vi "GET_ActiveData.vi"(8 "error in (no error)":errorcluster, 11 "FakedArray in":refnum<class "FakedArray.lvclass">) -> (0 "error out":errorcluster, 1 "Active Data []":i32[](array[numeric]), 2 "Path & Icon":T1, 3 "FakedArray out":refnum<class "FakedArray.lvclass">, 4 "Locked Layer":i32, 6 "Layer Locked?":bool)   [LabVIEW 2021, in "FakedArray.lvclass"]
uses:
  <resource>/plugins/NIIconEditor/Class/FakedArray/FakedArray.lvclass
  <vilib>/LabVIEW Icon API/lv_icon/Controls/Graphic.ctl
  <resource>/plugins/NIIconEditor/Class/FakedArray/FakedArray.lvclass/FakedArray.ctl
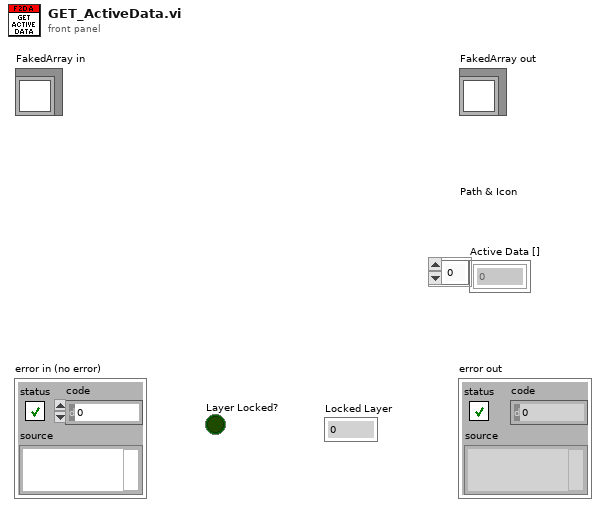
[diagram p1: front panel]
types:
  T1 = typedef "Graphic.ctl" = cluster{"Rectangle":cluster{"left":i16, "top":i16, "right":i16, "bottom":i16}, "Path":path, "Image":picture, "Filter":string, "FileName":string}
  T2 = typedef "ToMoreSpecific_Faked2DArray.ctl" = enum16{"Framework Templates", "Layer List"}
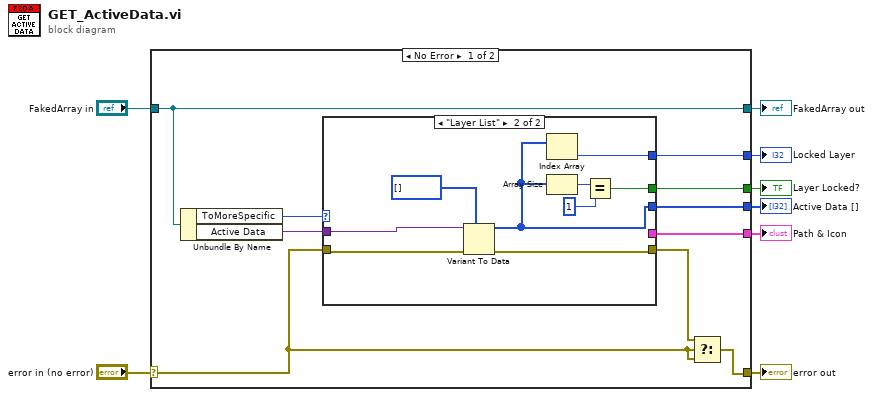
[diagram p0: block diagram]
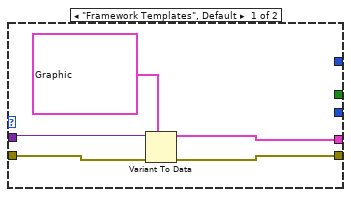
[diagram p2: hidden frame]
diagram:
  n1 = case shown="No Error" "error in (no error)" {
    selector: "error in (no error)" -> [w14 w34]
    tunnel: [w12 w34] -> w7
    tunnel: [w18 w33] -> w5
    tunnel: "FakedArray in" -> [w18 w33]
    tunnel: [w15 _] -> w4
    tunnel: [w11 _] -> w3
    tunnel: [w10 _] -> w2
    tunnel: [w9 _] -> w1
    frame No Error {
      n2 = Unbundle By Name(w18) -> ("ToMoreSpecific"=w17:T2, "Active Data"=w16:variant)
      n3 = case shown="\"Layer List\"" w17 {
        tunnel: w16 -> [w23 w32]
        tunnel: w14 -> [w22 w31]
        tunnel: [w21 w30] -> w13
        tunnel: [w19 _] -> w15
        tunnel: [_ w25] -> w11
        tunnel: [_ w26] -> w10
        tunnel: [_ w24] -> w9
        frame "Framework Templates", Default {
          n4 = Variant To Data(error in=w22, type=T1 {"Rectangle"={"left"=0, "top"=0, "right"=0, "bottom"=0}, "Path"=path "", "Image"=bytes[0], "Filter"="", "FileName"=""} ("Path & Icon"), Variant=w23) -> (data=w19:T1, error out=w21:errorcluster)
        }
        frame "Layer List" {
          n5 = Variant To Data(error in=w31, type=i32[] [], Variant=w32) -> (data=w25:i32[], error out=w30:errorcluster)
          n6 = Index Array(array=w25) -> (element=w24:i32)  [unwired: 1 in]
          n7 = Array Size(array=w25) -> (size(s)=w28:i32)
          n8 = Equal?(x=w28, y=1) -> (x = y?=w26:bool)
        }
      }
      n9 = Select(t=w13, s=w14, f=w14) -> (s? t:f=w12:errorcluster)
    }
    frame Error {
    }
  }
  "error out" <- w7
  "FakedArray out" <- w5
  "Path & Icon" <- w4
  "Active Data []" <- w3
  "Layer Locked?" <- w2
  "Locked Layer" <- w1
